vi "Drive Problem Fix.vi"(1 "Drive Global Data Modified":T1, 2 "Drive Global Data Original":T1) -> (0 "Drive Global Data New":T1)   [LabVIEW 2013]
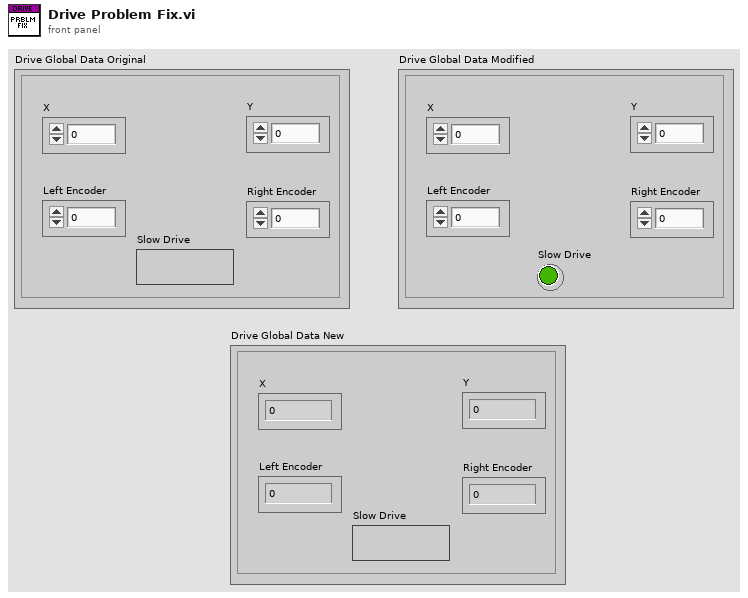
[diagram p1: front panel]
types:
  T1 = cluster{"Y":dbl, "X":dbl, "Left Encoder":dbl, "Right Encoder":dbl, "Slow Drive":bool}
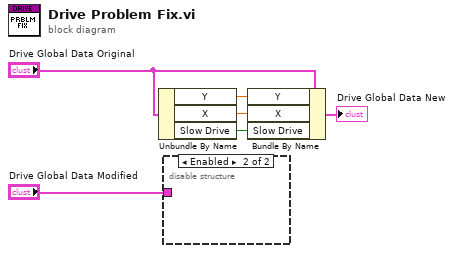
[diagram p0: block diagram]
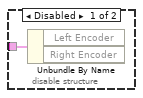
[diagram p2: hidden frame]
diagram:
  n1 = Unbundle By Name("Drive Global Data Original") -> ("Y"=w4:dbl, "X"=w3:dbl, "Slow Drive"=w1:bool)
  n2 = disable-structure shown="Enabled" {
    disable-tunnel: "Drive Global Data Modified" -> [w9 _]
    frame Disabled {
      n3 = Unbundle By Name(w9) -> ("Left Encoder"=w8:dbl, "Right Encoder"=w7:dbl)
    }
    frame Enabled {
    }
  }
  n4 = Bundle By Name(cluster="Drive Global Data Original", "Y"=w4, "X"=w3, "Slow Drive"=w1) -> (→"Drive Global Data New":T1)
